vi "write_loop_to_loop_fifo_flexRIO.vi"(5 "enable fly-back reversion?":bool, 6 "invert channels":bool[](array[boolean])=[FALSE, FALSE], 7 "fly-back?":bool, 8 "pixel finished?":bool, 10 "maximum bit depth":i8, 11 "integration cluster in":T1) -> (0 "local transfer FIFO full":bool, 3 "integration cluster out":T1)   [LabVIEW 2010]
uses:
  integration_cluster_flexRIO.ctl
  <vilib>/rvi/DataTransferAndStorage/Container/XNode/niFpgaContainer.xnode
  <vilib>/rvi/Memory/Memory_Emulation/nirvimemoryEmulationManagerCache_GetValue.vi
  <vilib>/rvi/DataTransferAndStorage/Container/Common/niFpgaContainerGetUniqueNameForEmu.vi
  <vilib>/rvi/Memory/Memory_Emulation/nirvimemoryEmulationManagerCache_InsertValue.vi
  <vilib>/Utility/error.llb/Clear Errors.vi
  <vilib>/rvi/Memory/Memory_Emulation/nirvimemoryEmulationManagerCache_SetValue.vi
  <vilib>/rvi/FIFO/Fifo_Resource/nirvififoEmulationSetSize.vi
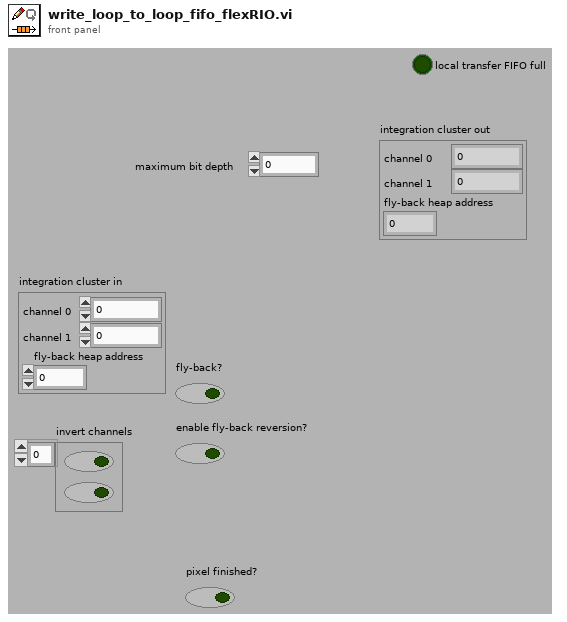
[diagram p1: front panel]
types:
  T1 = typedef "integration_cluster_flexRIO.ctl" = cluster{"channel 0":u32, "channel 1":u32, "fly-back heap address":u32}
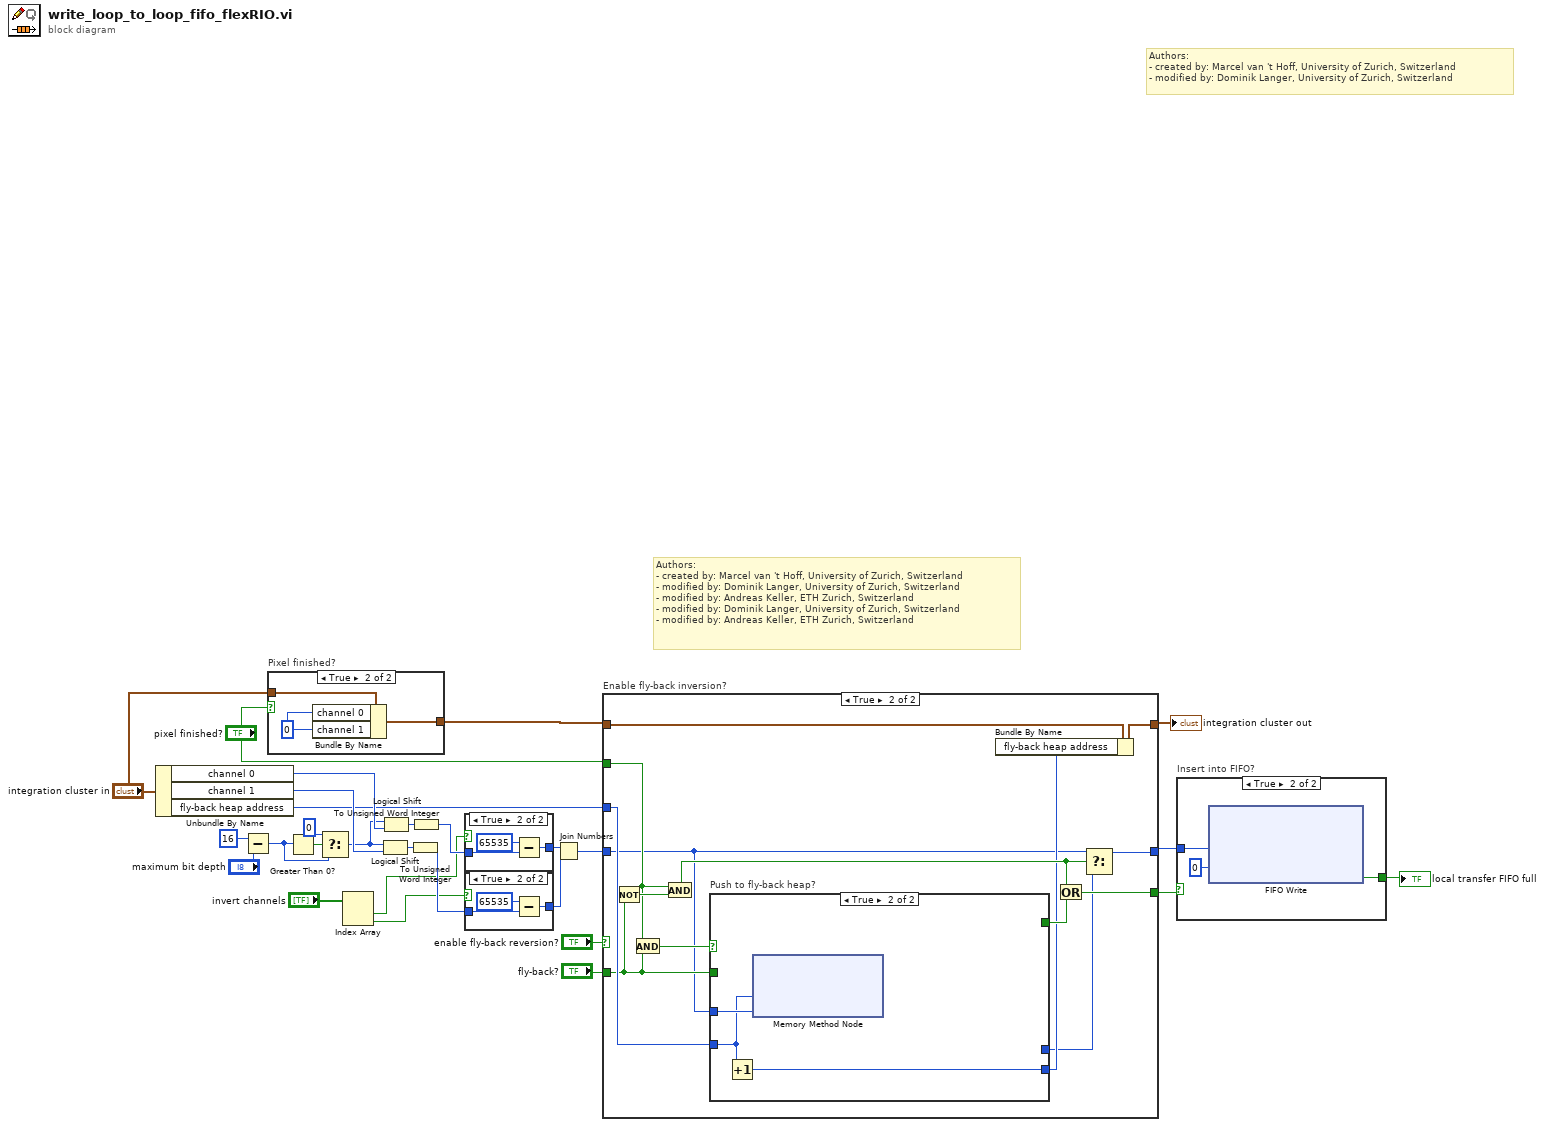
[diagram p0: block diagram]
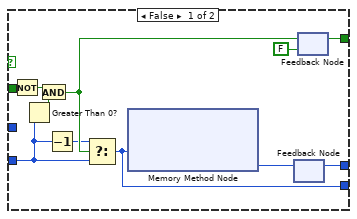
[diagram p6: hidden frame]
diagram:
  # "Authors: \n- created by: Marcel van 't Hoff, University of Zurich, Switzerland\n- modified by: Dominik Langer, University of Zurich, Switzerland\n- modified by: Andreas Keller, ETH Zurich, Switzerland\n- modified by: Dominik Langer, University of Zurich, Switzerland\n- modified by: Andreas Keller, ETH Zurich, Switzerland"
  # "Authors: \n- created by: Marcel van 't Hoff, University of Zurich, Switzerland\n- modified by: Dominik Langer, University of Zurich, Switzerland"
  n1 = Unbundle By Name("integration cluster in") -> ("channel 0"=w21:u32, "channel 1"=w22:u32, "fly-back heap address"=w13:u32)
  n2 = Subtract(x=i8 16, y="maximum bit depth") -> (x-y=w24:i8)
  n3 = case "Pixel finished?" shown="True" "pixel finished?" {
    tunnel: "integration cluster in" -> [w29 w31]
    tunnel: [w29 w30] -> w10
    frame False {
    }
    frame True {
      w32 = u32 0 ("channel 1")
      n4 = Bundle By Name(cluster=w31, "channel 0"=w32, "channel 1"=w32) -> (w30:T1)
    }
  }
  n5 = Greater Than 0?(x=w24) -> (x > 0?=w23:bool)
  n6 = Select(t=i8 0 ("f"), s=w23, f=w24) -> (s? t:f=w20:i8)
  n7 = Index Array(array="invert channels") -> (element #1=w2:bool, element #2=w1:bool)  [unwired: 2 in]
  n8 = Logical Shift(y=w20, x=w22) -> (x << y=w19:u32)
  n9 = Logical Shift(y=w20, x=w21) -> (x << y=w18:u32)
  n10 = To Unsigned Word Integer(number=w19) -> (unsigned 16bit integer=w5:u16)
  n11 = To Unsigned Word Integer(number=w18) -> (unsigned 16bit integer=w7:u16)
  n12 = case shown="True" w2 {
    tunnel: [w33 w35] -> w6
    tunnel: w7 -> [w33 w34]
    frame False {
    }
    frame True {
      n13 = Subtract(x=u16 65535, y=w34) -> (x-y=w35:u16)
    }
  }
  n14 = case shown="True" w1 {
    tunnel: [w37 w39] -> w4
    tunnel: w5 -> [w37 w38]
    frame False {
    }
    frame True {
      n15 = Subtract(x=u16 65535, y=w38) -> (x-y=w39:u16)
    }
  }
  n16 = Join Numbers(hi=w6, lo=w4) -> ((hi.lo)=w17:u32)
  n17 = case "Enable fly-back inversion?" shown="True" "enable fly-back reversion?" {
    tunnel: w13 -> [_ w57]
    tunnel: w17 -> [w43 w46]
    tunnel: [w43 w55] -> w16
    tunnel: "pixel finished?" -> [w42 w50]
    tunnel: [w42 w45] -> w12
    tunnel: "fly-back?" -> [_ w52]
    tunnel: w10 -> [w41 w49]
    tunnel: [w41 w47] -> w8
    frame False {
    }
    frame True {
      n18 = Not(x=w52) -> (.not. x?=w56:bool)
      n19 = And(x=w50, y=w52) -> (x .and. y?=w54:bool)
      n20 = And(x=w50, y=w56) -> (x .and. y?=w53:bool)
      n21 = case "Push to fly-back heap?" shown="True" w54 {
        tunnel: w46 -> [_ w197]
        tunnel: [w58 w196] -> w48
        tunnel: w57 -> [w60 w195]
        tunnel: w52 -> [w67 _]
        tunnel: [w63 _] -> w44
        tunnel: [w65 _] -> w51
        frame False {
          n22 = Not(x=w67) -> (.not. x?=w66:bool)
          n23 = Greater Than 0?(x=w60) -> (x > 0?=w68:bool)
          n24 = And(x=w66, y=w68) -> (x .and. y?=w61:bool)
          n25 = Decrement(x=w60) -> (x-1=w59:u32)
          n26 = Select(t=w59, s=w61, f=w60) -> (s? t:f=w58:u32)
          n27 = xnode ("Memory Method Node")("Address"=w58) -> ("Data"=w62:u32)  [unwired: 1 in, 1 out]
          n28 = feedback #1() -> (w63:u32)  [unwired: 1 in]
          n29 = feedback-in #1(w62) -> ()
          n30 = feedback #2(FALSE) -> (w65:bool)
          n31 = feedback-in #2(w61) -> ()
        }
        frame True {
          n32 = Increment(x=w195) -> (x+1=w196:u32)
          n33 = xnode ("Memory Method Node")("Address"=w195, "Data"=w197) -> ()  [unwired: 1 in, 1 out]
        }
      }
      n34 = Bundle By Name(cluster=w49, "fly-back heap address"=w48) -> (w47:T1)
      n35 = Or(x=w53, y=w51) -> (x .or. y?=w45:bool)
      n36 = Select(t=w46, s=w53, f=w44) -> (s? t:f=w55:u32)
    }
  }
  "integration cluster out" <- w8
  n37 = case "Insert into FIFO?" shown="True" w12 {
    tunnel: [_ w325] -> w27
    tunnel: w16 -> [_ w323]
    frame False {
    }
    frame True {
      n38 = xnode ("FIFO Write")("Element"=w323, "Timeout"=0) -> ("Timed Out?"=w325:bool)  [unwired: 1 in, 1 out]
    }
  }
  "local transfer FIFO full" <- w27
